vi "_io_read_chunked_timeout.vi"(7 "Timeout in":i32, 8 "error in":errorcluster caption="error in (no error)", 9 "Allow Assure End with LF":bool=TRUE, 10 "Max bytes to read":u32, 11 "VISA resource name":refnum<visa-resource-name>) -> (0 "error out":errorcluster, 1 "Read bytes count":i32, 2 "Read buffer":string, 3 "VISA resource name out":refnum<visa-resource-name>, 4 "TimedOut":bool)   [LabVIEW 2022 SP3, in "hmp4000_rsidr_core.lvlib"]
doc: "Same functionality as VISA Read, but with one difference:\nVISA read timeout is set to maximum of 5000 ms, and more VISA Reads are stacked one after another until either a response comes, or the entered timeout expires.\nRather than entering long VISA timeouts, this makes the LabVIEW application more responsive, because the maximum time when your program is non-responsive is capped to 5000 ms."
uses:
  hmp4000_rsidr_core.lvlib
  type_Error_Codes.ctl
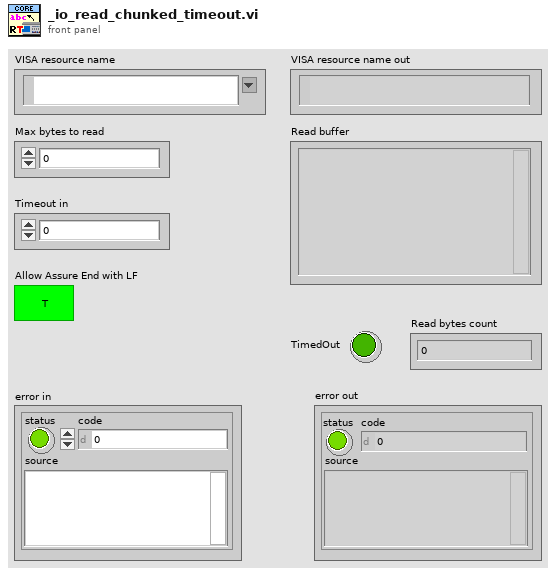
[diagram p1: front panel]
types:
  T1 = typedef "hmp4000_rsidr_core.lvlib/type_Error_Codes.ctl" = enum16{"No_error", "VISA_err_ResourceNotFound", "VISA_err_Timeout", "VISA_warn_MoreDataAvailable", "RS_err_MissingCallback", "RS_err_InvalidAttribute", "RS_err_InvalidValue", "RS_err_UnknownResource", "RS_err_AlreadyInitialized", "RS_err_InstrumentStatus", "RS_err_BadRepCapName", "RS_err_TypesMismatch", "RS_err_ValueNotSupported", "RS_err_InvalidRngTable", "RS_err_IDqueryFail", "RS_err_UnexpResponse", "VISA_warn_ConfigNotLoaded", "RS_err_AttributeNotReadable", "RS_err_AttributeNotWritable", "RS_err_InstrumentType", "RS_err_InstrumentOption", "VISA_err_InvalidSize", "RS_err_ReliabilityIndicator", "VISA_warn_UnknownStatus", "VISA_warn_TermCharRead", "VISA_err_IO_error", "RS_err_FunctionNotSupported", "VISA_warn_QueueEmpty"}
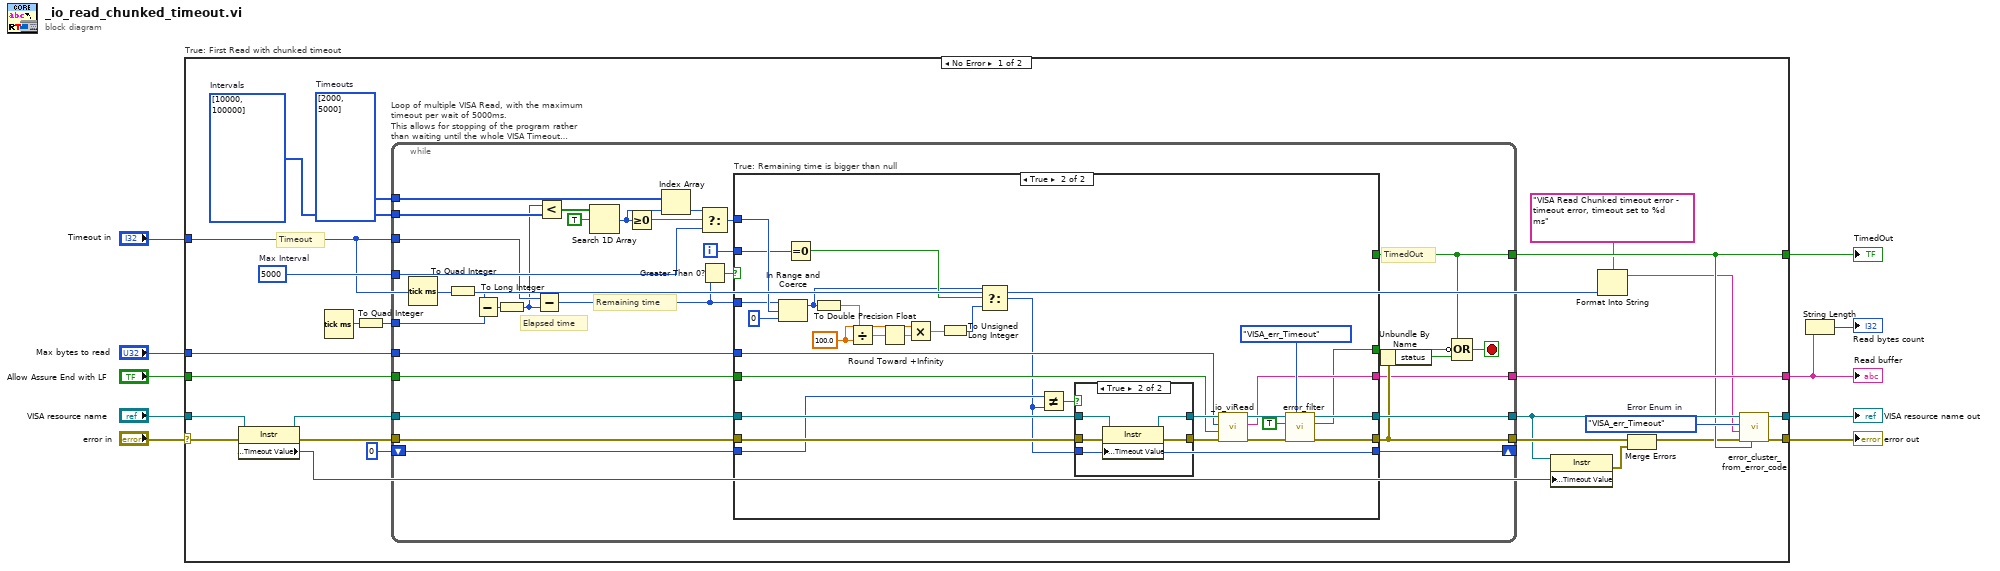
[diagram p0: block diagram]
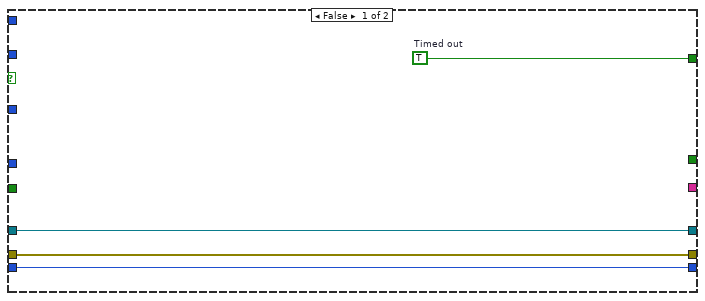
[diagram p2: hidden frame]
diagram:
  n1 = case "True: First Read with chunked timeout" shown="No Error" "error in" {
    selector: "error in" -> [w12 w108]
    tunnel: "VISA resource name" -> [w16 w107]
    tunnel: [w25 w107] -> w2
    tunnel: "Timeout in" -> [w21 _]
    tunnel: [w29 _] -> w5
    tunnel: "Max bytes to read" -> [w28 _]
    tunnel: [w24 w108] -> w3
    tunnel: [w23 _] -> w6
    tunnel: "Allow Assure End with LF" -> [w11 _]
    frame No Error {
      w27 = type_Error_Codes."VISA_err_Timeout"  # Error Enum in
      w31 = i64 5000  # Max Interval
      w33 = i32[] [2000, 5000]  # Timeouts
      w34 = i64[] [10000, 100000]  # Intervals
      # "Timeout"
      n2 = property on="Property Node" class="Instr"(reference=w16, error in=w12) -> (reference out=w14:refnum<visa-resource-name>, error out=w15:errorcluster, "General Settings:Timeout Value"=w13:u32)
      n3 = Tick Count (ms)() -> (millisecond timer value=w32:u32)
      n4 = To Quad Integer(1:w32) -> (0:w17:i64)
      n5 = while "Loop of multiple VISA Read, with the maximum timeout per wait of 5000ms.\nThis allows for stopping of the program rather than waiting until the whole VISA Timeout expires" {
        tunnel: w33 -> [w61]
        tunnel: w31 -> [w52]
        tunnel: w34 -> [w60]
        tunnel: w15 -> [w59]
        tunnel: w14 -> [w58]
        tunnel: [w50] -> w35
        tunnel: [w57] -> w26
        tunnel: w21 -> [w47]
        tunnel: [w46] -> w29
        tunnel: w28 -> [w44]
        tunnel: [w43] -> w23
        shift-right: [w41] -> _
        shift-left: u32 0 -> [w40]
        tunnel: w17 -> [w39]
        tunnel: w11 -> [w36]
        i -> [w37]
        stop <- w48 stop-if-true
        # "Remaining time"
        # "TimedOut"
        # "Elapsed time"
        n6 = Tick Count (ms)() -> (millisecond timer value=w56:u32)
        n7 = To Quad Integer(1:w56) -> (0:w45:i64)
        n8 = Subtract(x=w45, y=w39) -> (x-y=w55:i64)
        n9 = To Long Integer(number=w55) -> (32bit integer=w38:i32)
        n10 = Subtract(x=w47, y=w38) -> (x-y=w51:i32)
        n11 = Less?(x=w38, y=w60) -> (x < y?=w66:bool[])
        n12 = Search 1D Array(1D array=w66, element=TRUE) -> (index of element=w63:i32)  [unwired: 1 in]
        n13 = Greater Or Equal To 0?(x=w63) -> (x >= 0?=w64:bool)
        n14 = Index Array(array=w61, index=w63) -> (element=w62:i32)
        n15 = Select(t=w62, s=w64, f=w52) -> (s? t:f=w53:i64)
        n16 = Greater Than 0?(x=w51) -> (x > 0?=w54:bool)
        n17 = case "True: Remaining time is bigger than null" shown="True" w54 {
          tunnel: w59 -> [w70 w92]
          tunnel: w58 -> [w69 w90]
          tunnel: [w70 w87] -> w50
          tunnel: [w69 w88] -> w57
          tunnel: w51 -> [_ w98]
          tunnel: w53 -> [_ w99]
          tunnel: [w68 _] -> w43
          tunnel: [_ w86] -> w46
          tunnel: w44 -> [_ w85]
          tunnel: [_ w84] -> w42
          tunnel: [w67 w71] -> w41
          tunnel: w40 -> [w67 w82]
          tunnel: w37 -> [_ w76]
          tunnel: w36 -> [_ w72]
          frame False {
            w68 = TRUE  # Timed out
          }
          frame True {
            w79 = 100.0 ("y")
            n18 = In Range and Coerce(upper limit=w98, x=w99, lower limit=i64 0) -> (coerced(x)=w74:i64)  [unwired: 1 out]
            n19 = Equal To 0?(x=w76) -> (x = 0?=w75:bool)
            n20 = To Double Precision Float(number=w74) -> (double precision float=w77:dbl)
            n21 = Divide(x=w77, y=w79) -> (x/y=w81:dbl)
            n22 = Round Toward +Infinity(x=w81) -> (ceil(x): smallest int >= x=w80:dbl)
            n23 = Multiply(x=w79, y=w80) -> (x*y=w78:dbl)
            n24 = To Unsigned Long Integer(number=w78) -> (unsigned 32bit integer=w73:u32)
            n25 = Select(t=w74, s=w75, f=w73) -> (s? t:f=w71:i64)
            n26 = Not Equal?(x=w82, y=w71) -> (x != y?=w83:bool)
            n27 = case shown="True" w83 {
              tunnel: w92 -> [w101 w106]
              tunnel: [w101 w105] -> w91
              tunnel: w71 -> [_ w104]
              tunnel: w90 -> [w100 w103]
              tunnel: [w100 w102] -> w89
              frame False {
              }
              frame True {
                n28 = property on="Property Node" class="Instr"(reference=w103, error in=w106, "General Settings:Timeout Value"=w104) -> (reference out=w102:refnum<visa-resource-name>, error out=w105:errorcluster)
              }
            }
            n29 = call "_io_viRead.vi"("error in"=w91, "Allow Assure End with LF"=w72, "Max bytes to read"=w85, "VISA resource name"=w89) -> ("error out"=w94:errorcluster, "Read buffer"=w86:string, "VISA resource name out"=w93:refnum<visa-resource-name>)  [unwired: 4 in, 1 out]
            n30 = call "error_filter.vi"("Error Enum in"=type_Error_Codes."VISA_err_Timeout", "error in"=w94, "Clear detected code (F)"=TRUE ("Clear detected code"), "VISA resource name"=w93) -> ("error out"=w87:errorcluster, "Code Detected"=w84:bool, "VISA resource name out"=w88:refnum<visa-resource-name>)  [unwired: 5 in]
          }
        }
        n31 = Unbundle By Name(w50) -> ("status"=w49:bool)
        n32 = Compound Arithmetic op=OR(w43, invert w42, w49) -> (w48:bool)
      }
      n33 = property on="Property Node" class="Instr"(reference=w26, "General Settings:Timeout Value"=w13) -> (error out=w30:errorcluster)  [unwired: 1 in, 1 out]
      n34 = Format Into String(format string="VISA Read Chunked timeout error - timeout error, timeout set to %d ms", w21) -> (resulting string=w20:string)  [unwired: 2 in, 1 out]
      n35 = Merge Errors(w35, w30) -> (w19:errorcluster)
      n36 = call "error_cluster_from_error_code.vi"("Error Creation Enabled (True)"=w23, "error in"=w19, "Error Message (\"\")"=w20, "Error Enum in"=w27, "VISA resource name"=w26) -> ("error out"=w24:errorcluster, "VISA resource name out"=w25:refnum<visa-resource-name>)  [unwired: 5 in]
    }
    frame Error {
    }
  }
  "TimedOut" <- w6
  "Read buffer" <- w5
  "VISA resource name out" <- w2
  "error out" <- w3
  n37 = String Length(string=w5) -> (length=→"Read bytes count":i32)
